vi "Batch SPARC 3.1.vi"(8 "Error In":errorcluster) -> (0 "Error Out":errorcluster, 3 "Saved Path":string)   [LabVIEW 2020]
uses:
  <userlib>/_OpenG.lib/file/file.llb/File Exists - Scalar__ogtk.vi
  <vilib>/regexp/Match Regular Expression.xnode
panel:
  out "Settings Tested":u8(slide) scale=0.007..1.0
  out "Files Searched":u8(slide) scale=0.007..2.0
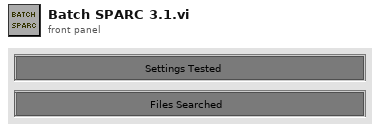
[diagram p1: front panel]
types:
  T1 = enum16{"open", "replace", "create", "open or create", "replace or create", "replace or create with confirmation"}
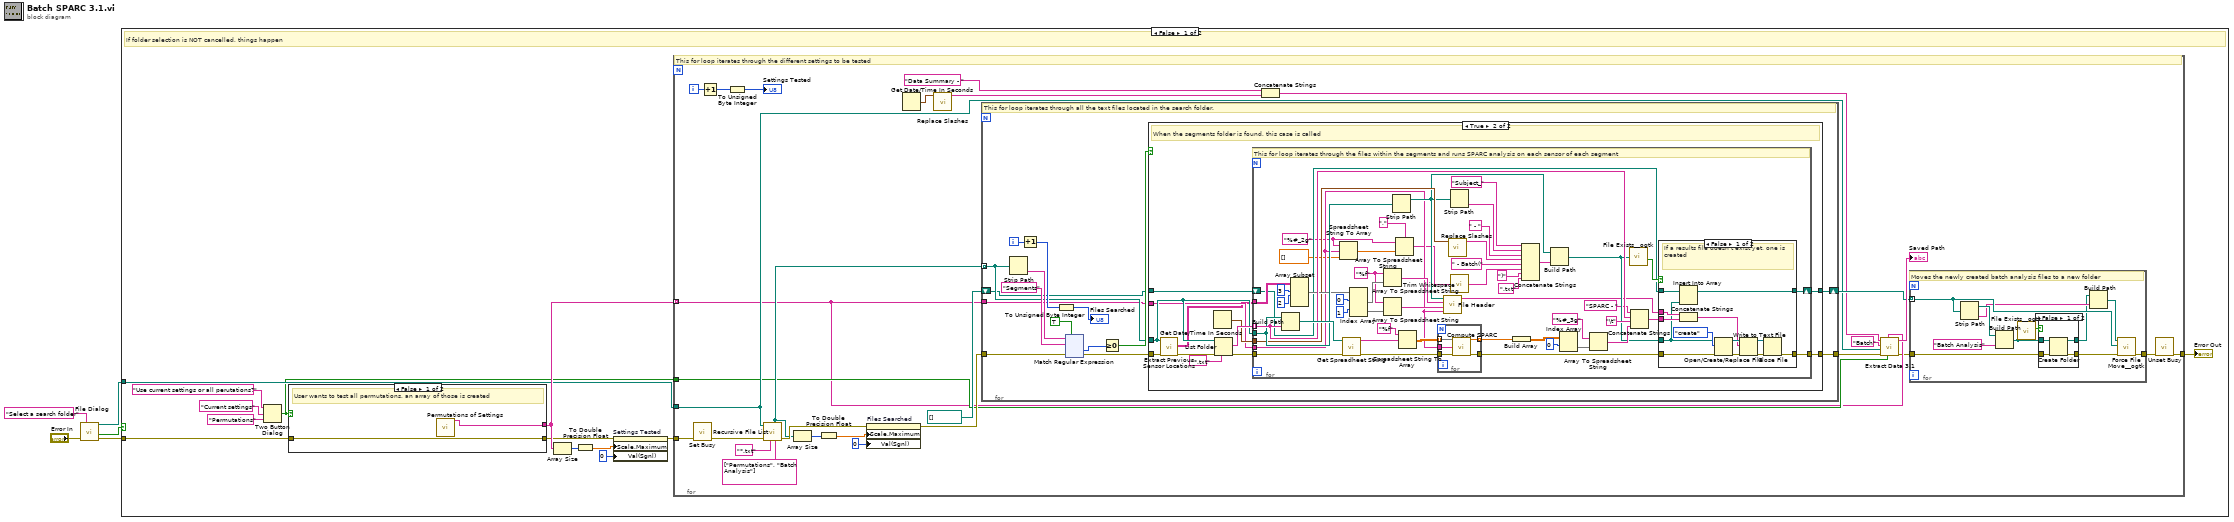
[diagram p0: block diagram]
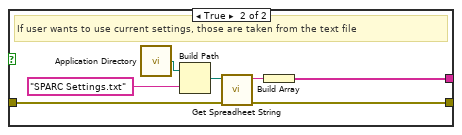
[diagram p2: hidden frame]
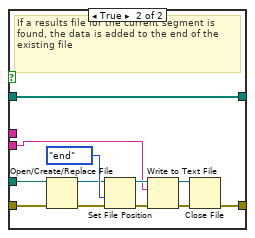
[diagram p5: hidden frame]
diagram:
  n1 = call "File Dialog"("prompt"="Select a search folder", "error in"="Error In") -> ("selected path"=w4:path, "cancelled"=w2:bool, "error out"=w3:errorcluster)  [unwired: 10 in, 1 out]
  n2 = case shown="False" w2 {
    tunnel: w4 -> [w8 _]
    tunnel: w3 -> [w17 _]
    frame False {
      # "If folder selection is NOT cancelled, things happen"
      n3 = Two Button Dialog(message="Use current settings or all perutations?", 1:"Permutations" ("F button name (\"Cancel\")"), 2:"Current settings" ("T button name (\"OK\")")) -> (T button?=w6:bool)
      n4 = case shown="False" w6 {
        tunnel: w17 -> [w19 w24]
        tunnel: [w19 w23] -> w7
        tunnel: [w20 w21] -> w14
        frame False {
          # "User wants to test all permutations, an array of those is created"
          n5 = call "Permutations of Settings.vi"() -> ("Settings Permutations"=w20:string[])  [unwired: 11 in]
        }
        frame True {
          # "If user wants to use current settings, those are taken from the text file"
          n6 = call <vilib>:"Application Directory.vi"() -> ("Application Directory"=w26:path)
          n7 = Build Path(base path=w26, name or relative path="SPARC Settings.txt") -> (appended path=w27:path)
          n8 = call "Get Spreadheet String.vi"("error in (no error)"=w24, "File Path"=w27) -> ("error out"=w23:errorcluster, "Spreadsheet String"=w22:string)  [unwired: 8 in]
          n9 = Build Array(w22) -> (w21:string[])
        }
      }
      n10 = Array Size(array=w14) -> (size(s)=w13:i32)
      n11 = To Double Precision Float(number=w13) -> (double precision float=w12:dbl)
      n12 = property on="Settings Tested" class="Slide (strict)"(error in=w7, "Scale.Maximum"=w12, "Val(Sgnl)"=u8 0 ("Value (Signaling)")) -> (error out=w16:errorcluster)  [unwired: 1 in, 1 out]
      n13 = for {
        tunnel: w8 -> [w33]
        tunnel: w16 -> [w54]
        tunnel: [w44] -> w18
        tunnel: w14 -> [w31] mode=indexing
        tunnel: w6 -> [w32]
        i -> [w37]
        # "This for loop iterates through the different settings to be tested"
        n14 = call <vilib>:"Set Busy.vi"("error in (no error)"=w54) -> ("error out"=w53:errorcluster)  [unwired: 9 in, 1 out]
        n15 = Increment(x=w37) -> (x+1=w36:i32)
        n16 = To Unsigned Byte Integer(number=w36) -> (unsigned 8bit integer=→"Settings Tested":u8)
        n17 = call <vilib>:"Recursive File List.vi"("Folders to Exclude"=string[] ["Permutations", "Batch Analysis"], "pattern"="*.txt", "error in (no error)"=w53, "Folder Path"=w33) -> ("error out"=w52:errorcluster, "All Folders"=w48:path[])  [unwired: 3 in, 3 out]
        n18 = Array Size(array=w48) -> (size(s)=w51:i32)
        n19 = To Double Precision Float(number=w51) -> (double precision float=w50:dbl)
        n20 = property on="Files Searched" class="Slide (strict)"(error in=w52, "Scale.Maximum"=w50, "Val(Sgnl)"=u8 0 ("Value (Signaling)")) -> (error out=w49:errorcluster)  [unwired: 1 in, 1 out]
        n21 = Get Date/Time In Seconds() -> (seconds since 1Jan1904=w41:timestamp)
        n22 = call "Replace Slashes.vi"("time stamp"=w41) -> ("Date & Time String"=w40:string)  [unwired: 10 in]
        n23 = for {
          tunnel: w48 -> [w76] mode=indexing
          tunnel: w49 -> [w87]
          tunnel: [w78] -> w30
          shift-right: [w74] -> w43
          shift-left: path[] [] -> [w75]
          tunnel: w31 -> [w73]
          i -> [w84]
          # "This for loop iterates through all the text files located in the search folder."
          n24 = Strip Path(path=w76) -> (name=w77:string)  [unwired: 1 out]
          n25 = Increment(x=w84) -> (x+1=w85:i32)
          n26 = To Unsigned Byte Integer(number=w85) -> (unsigned 8bit integer=→"Files Searched":u8)
          n27 = xnode "Match Regular Expression"("input string"=w77, "regular expression"="Segments", "error in"=w87, "ignore case? (F)"=TRUE) -> ("offset past match"=w80:i32, "error out"=w79:errorcluster)  [unwired: 2 in, 3 out]
          n28 = Greater Or Equal To 0?(x=w80) -> (x >= 0?=w83:bool)
          n29 = case shown="True" w83 {
            tunnel: w79 -> [w203 w209]
            tunnel: w76 -> [_ w211]
            tunnel: [w203 w215] -> w78
            tunnel: w75 -> [w202 w206]
            tunnel: [w202 w207] -> w74
            tunnel: w73 -> [_ w205]
            frame False {
              # "When the iteration of the search files is not within the segments folder, nothing happens."
            }
            frame True {
              # "When the segments folder is found, this case is called"
              n30 = call "Extract Previous Sensor Locations.vi"("error in (no error)"=w209, "Folder Path"=w211) -> ("error out"=w210:errorcluster, "Smoothness Exam Text"=w204:string[][])  [unwired: 7 in, 1 out]
              n31 = Get Date/Time In Seconds() -> (seconds since 1Jan1904=w208:timestamp)
              n32 = List Folder(path=w211, pattern="*.txt", error in=w210) -> (filenames=w212:string[], error out=w213:errorcluster)  [unwired: 1 in, 2 out]
              n33 = for {
                tunnel: w212 -> [w252] mode=indexing
                tunnel: w213 -> [w267]
                tunnel: [w251] -> w215
                tunnel: w211 -> [w250]
                tunnel: w204 -> [w248]
                tunnel: w208 -> [w237]
                shift-right: [w229] -> w207
                shift-left: w206 -> [w228]
                tunnel: w205 -> [w222]
                w219 = "%#_2g" ("format string")
                w238 = "%f" ("format string")
                # "This for loop iterates through the files within the segments and runs SPARC analysis on each sensor of each segment"
                n34 = Build Path(base path=w250, name or relative path=w252) -> (appended path=w263:path)
                n35 = Array Subset(array=w248, index (row)=3 ("index"), length (row)=2 ("length")) -> (w245:string[][])  [unwired: 2 in]
                n36 = Spreadsheet String To Array(format string=w219, spreadsheet string=w222, array type (2D Dbl)=dbl[] []) -> (array=w220:dbl[])  [unwired: 1 in]
                n37 = call "Get Spreadheet String.vi"("error in (no error)"=w267, "File Path"=w263) -> ("error out"=w226:errorcluster, "Spreadsheet String"=w265:string)  [unwired: 8 in]
                n38 = Index Array(array=w245, index (row) #1=0 ("index (row)"), index (row) #2=1 ("index (row)")) -> (element #1=w239:string[], element #2=w240:string[])  [unwired: 2 in]
                n39 = Array To Spreadsheet String(array=w239, 3:w238) -> (spreadsheet string=w242:string)  [unwired: 1 in]
                n40 = Array To Spreadsheet String(array=w240, 3:w238) -> (spreadsheet string=w241:string)  [unwired: 1 in]
                n41 = Strip Path(path=w250) -> (stripped path=w232:path)  [unwired: 1 out]
                n42 = Array To Spreadsheet String(delimiter (Tab)="," ("string"), array=w220, 3:w219) -> (spreadsheet string=w217:string)
                n43 = Spreadsheet String To Array(format string="%f", spreadsheet string=w265) -> (array=w264:dbl[][])  [unwired: 2 in]
                n44 = for {
                  tunnel: [w296] -> w231
                  tunnel: [w297] -> w254 mode=indexing
                  tunnel: w264 -> [w293] mode=indexing
                  tunnel: w222 -> [w294]
                  tunnel: w226 -> [w295]
                  n45 = call "Compute SPARC.vi"("Pressure Array"=w293, "Settings"=w294, "error in"=w295) -> ("SPARC"=w297:dbl, "error out"=w296:errorcluster)  [unwired: 11 in]
                }
                n46 = call "File Header.vi"("Settings"=w222, "Sensors"=w241, "Locations"=w242, "Stripped Path"=w232) -> ("File Header"=w225:string)  [unwired: 7 in]
                n47 = call "Replace Slashes.vi"("time stamp"=w237) -> ("Date & Time String"=w227:string)  [unwired: 10 in]
                n48 = Strip Path(path=w232) -> (name=w234:string)  [unwired: 1 out]
                n49 = call <vilib>:"Trim Whitespace.vi"("string"=w217) -> ("trimmed string"=w216:string)  [unwired: 1 in]
                n50 = Build Array(w254) -> (w253:dbl[][])
                n51 = Concatenate Strings("Subject_" ("string"), w234, " - " ("string"), w227, " - Batch(" ("string"), w216, ")" ("string"), ".txt" ("string")) -> (w260:string)
                n52 = Build Path(base path=w232, name or relative path=w260) -> (appended path=w249:path)
                n53 = Index Array(array=w253, index (row)=0) -> (element=w261:dbl[])  [unwired: 1 in]
                n54 = Array To Spreadsheet String(array=w261, 3:"%#_3g" ("format string")) -> (spreadsheet string=w259:string)  [unwired: 1 in]
                n55 = call-poly <userlib>:"File Exists__ogtk.vi"("file path"=w249) -> ("exists"=w262:bool)  [unwired: 6 in, 1 out]
                n56 = Concatenate Strings("SPARC - " ("string"), w252, "\t", w259) -> (w258:string)
                n57 = case shown="False" w262 {
                  tunnel: w225 -> [w274 _]
                  tunnel: w249 -> [w269 w292]
                  tunnel: [w276 w286] -> w251
                  tunnel: w258 -> [w272 w283]
                  tunnel: w231 -> [w271 w282]
                  tunnel: w228 -> [w270 w281]
                  tunnel: [w268 w281] -> w229
                  frame False {
                    # "If a results file doesn't exist yet, one is created"
                    n58 = Concatenate Strings(w274, w272) -> (w273:string)
                    n59 = Insert Into Array(array=w270, new element=w269) -> (w268:path[])  [unwired: 1 in]
                    n60 = Open/Create/Replace File(file path (use dialog)=w269, error in=w271, operation (0:open)=T1."create") -> (refnum out=w279:refnum<file>, error out=w278:errorcluster)  [unwired: 3 in, 1 out]
                    n61 = Write to Text File(file (use dialog)=w279, text=w273, error in=w278) -> (refnum out=w275:refnum<file>, error out=w277:errorcluster)  [unwired: 1 in, 1 out]
                    n62 = Close File(refnum=w275, error in=w277) -> (error out=w276:errorcluster)  [unwired: 1 out]
                  }
                  frame True {
                    # "If a results file for the current segment is found, the data is added to the end of the existing file"
                    n63 = Open/Create/Replace File(file path (use dialog)=w292, error in=w282) -> (refnum out=w290:refnum<file>, error out=w289:errorcluster)  [unwired: 4 in, 1 out]
                    n64 = Set File Position(refnum=w290, from (0:start)=enum16{"start", "end", "current"}."end", error in=w289) -> (refnum out=w285:refnum<file>, error out=w288:errorcluster)  [unwired: 1 in]
                    n65 = Write to Text File(file (use dialog)=w285, text=w283, error in=w288) -> (refnum out=w284:refnum<file>, error out=w287:errorcluster)  [unwired: 1 in, 1 out]
                    n66 = Close File(refnum=w284, error in=w287) -> (error out=w286:errorcluster)  [unwired: 1 out]
                  }
                }
              }
            }
          }
        }
        n67 = Concatenate Strings("Data Summary - " ("Summary File Title"), w40) -> (w39:string)
        n68 = call "Extract Data 3.1.vi"("Single/Permutations"=w32, "Settings"=w31, "Error In"=w30, "Search Path"=w33, "File Search Phrase"="Batch", "Summary File Title"=w39) -> ("error out"=w29:errorcluster, "Saved Path"=→"Saved Path":string)  [unwired: 4 in]
        n69 = for {
          tunnel: w43 -> [w61] mode=indexing
          tunnel: w29 -> [w62]
          tunnel: [w59] -> w28
          # "Moves the newly created batch analysis files to a new folder"
          n70 = Strip Path(path=w61) -> (stripped path=w66:path, name=w57:string)
          n71 = Build Path(base path=w66, name or relative path="Batch Analysis") -> (appended path=w63:path)
          n72 = call-poly <userlib>:"File Exists__ogtk.vi"("file path"=w63) -> ("is directory"=w64:bool)  [unwired: 6 in, 1 out]
          n73 = case shown="False" w64 {
            tunnel: w63 -> [w70 w71]
            tunnel: w62 -> [w69 w72]
            tunnel: [w68 w72] -> w60
            tunnel: [w67 w71] -> w56
            frame False {
              n74 = Create Folder(path (use dialog)=w70, error in=w69) -> (created path=w67:path, error out=w68:errorcluster)  [unwired: 1 in, 1 out]
            }
            frame True {
            }
          }
          n75 = Build Path(base path=w56, name or relative path=w57) -> (appended path=w58:path)
          n76 = call <userlib>:"Force File Move__ogtk.vi"("error in (no error)"=w60, "source"=w61, "target"=w58) -> ("error out"=w59:errorcluster)  [unwired: 3 in, 1 out]
        }
        n77 = call <vilib>:"Unset Busy.vi"("error in (no error)"=w28) -> ("error out"=w44:errorcluster)  [unwired: 10 in]
      }
      "Error Out" <- w18
    }
    frame True {
      # "If file selection is cancelled, nothing happens."
    }
  }
